vi "Fetch Unit Data.vi"(8 "error in (no error)":errorcluster, 9 "End Channel (1)":string="0001", 10 "Start Channel (1)":string="0001", 11 "VISA resource name":refnum<visa-resource-name>) -> (0 "error out":errorcluster, 1 "Unit":string[](array[string]), 2 "Channel":string[](array[string]), 3 "VISA resource name out":refnum<visa-resource-name>, 4 "Decimal Position":i32[](array[numeric]), 5 "Data Status":i32[](array[numeric]))   [LabVIEW 2020, in "Yokogawa GX Series.lvlib"]
doc: "Reads the channel number, data status, decimal position, and unit."
uses:
  <instrlib>/Yokogawa GX Series/Yokogawa GX Series.lvlib
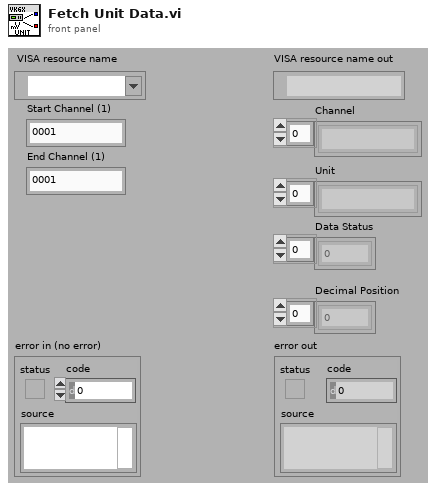
[diagram p1: front panel]
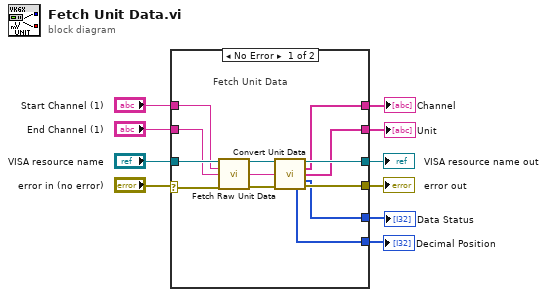
[diagram p0: block diagram]
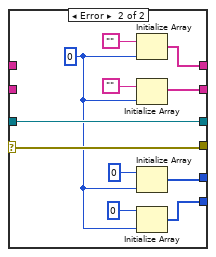
[diagram p2: hidden frame]
diagram:
  n1 = case shown="No Error" "error in (no error)" {
    selector: "error in (no error)" -> [w11 w33]
    tunnel: "VISA resource name" -> [w23 w34]
    tunnel: [w21 w34] -> w9
    tunnel: [w19 w33] -> w8
    tunnel: "Start Channel (1)" -> [w18 _]
    tunnel: "End Channel (1)" -> [w17 _]
    tunnel: [w15 w31] -> w4
    tunnel: [w14 w28] -> w2
    tunnel: [w13 w26] -> w1
    tunnel: [w12 w29] -> w3
    frame No Error {
      # "Fetch Unit Data"
      n2 = call <instrlib>:"Fetch Raw Unit Data.vi"("VISA resource name"=w23, "Start Channel (1)"=w18, "End Channel (1)"=w17, "error in (no error)"=w11) -> ("VISA resource name out"=w22:refnum<visa-resource-name>, "Unit Data"=w16:string, "error out"=w20:errorcluster)  [unwired: 9 out]
      n3 = call <instrlib>:"Convert Unit Data.vi"("VISA resource name"=w22, "Unit Data (\"\")"=w16, "error in (no error)"=w20) -> ("VISA resource name out"=w21:refnum<visa-resource-name>, "Channel"=w15:string[], "Unit"=w12:string[], "Data Status"=w14:i32[], "Decimal Position"=w13:i32[], "error out"=w19:errorcluster)  [unwired: 7 out]
    }
    frame Error {
      w24 = 0
      n4 = Initialize Array("", w24) -> (w31:string[])
      n5 = Initialize Array("", w24) -> (w29:string[])
      n6 = Initialize Array(0, w24) -> (w28:i32[])
      n7 = Initialize Array(0, w24) -> (w26:i32[])
    }
  }
  "error out" <- w8
  "VISA resource name out" <- w9
  "Channel" <- w4
  "Unit" <- w3
  "Data Status" <- w2
  "Decimal Position" <- w1
